vi "ecg_ncs_v9.vi"() -> ()   [LabVIEW 2016]
uses:
  <instrlib>/niUSRP/niUSRP Timestamp.ctl
  C:/Program Files/National Instruments/LabVIEW 2016/examples/Instrument IO/Serial/support/Serial - Settings.ctl
  State.ctl
  <vilib>/Instr/_visa.llb/VISA Configure Serial Port (Instr).vi
  <instrlib>/niUSRP/niUSRP Fetch Rx Data (2D CDB).vi
  <instrlib>/niUSRP/niUSRP Write Tx Data (2D CDB).vi
panel:
  out "#NCS Loops":i32
  out "size(s) 3":i32
  out "AmpNcsDSLast":dbl[](array[numeric])
  in  "Low-Pass Freq":dbl=200.0 format="%#_13g"
  in  "Wait  ECG":i32=2
  in  "max queue size":i32=-1
  in  "Wait NCS":i32=8
  out "ECG time":u32
  out "NCS time":u32
  in  "File Name 3":string="Test2"
  out "size(s) 4":i32
  in  "maxWrite 2":i32=2000
  out "AmpNcs":dbl[](array[numeric])
  out "PhNcs":dbl[](array[numeric])
  in  "Sampling Rate":i32=500
  out "AmpNcsDS":dbl[](array[numeric])
  out "PhNcsDS":dbl[](array[numeric])
  in  "Tab Control 3":enum32{"ECG Sample", "ECG"}(tab)
  out "?":i32(graph)
  out "?":i16(graph)
  in  "maxWrite":i32=2000
  out "size(s) 2":i32
  out "sizeNcsDS":i32
  in  "File Name":string="data"
  in  "Path":path=path "D:/Research/SummerFall17Spring18/CnC/NCS/EcgNcsCorrelation/CodeAndData/Data"
  out "#Loop = #Packets Received":i32
  out "ECGsample":i16
  out "error IO 2":errorcluster={"status"=FALSE, "code"=-1074118647, "source"=""}
  in  "Serial Settings":T1={"baud rate"=57600, "data bits"=8, "parity"=enum."None", "stop bits"=10, "flow control"=0} {"flow control" items=["None"=0, "XON/XOFF"=1, "RTS/CTS"=2, "DTR/DSR"=4]; "stop bits" items=["1.0"=10, "1.5"=15, "2.0"=20]; "data bits" min=5 max=8 step=1; "baud rate" items=["75"=75, "110"=110, "134"=134, "150"=150, "300"=300, "600"=600, "1200"=1200, "1800"=1800, "2400"=2400, "4800"=4800, "7200"=7200, "9600"=9600, "14400"=14400, "19200"=19200, "28800"=28800, "38400"=38400, "56000"=56000, "57600"=57600, "115200"=115200, "128000"=128000, "230400"=230400]}
  in  "VISA resource name":refnum<visa-resource-name>="bmd101"
  in  "byte count":u32=1
  out "Coerced Rx IQ Rate":dbl
  out "Gain":dbl=-15.0
  out "Bandwidth":dbl=56000000.0
  out "Coerced Carrier Frequency":dbl=2000000000.0 format="%#.17g"
  out "Coerced Tx IQ rate":dbl=1000000.0
  out "error IO":errorcluster={"status"=FALSE, "code"=-1074118647, "source"=""}
  in  "Rx Number of Samples":i32=2000
  in  "Tab Control 2":enum32{"NI-294x/295x", "NI-2900/2901"}(tab)=enum."NI-2900/2901"
  in  "Rx carrier frequency [Hz]":dbl=2000000000.0 format="%#_6p"
  in  "Tx carrier frequency [Hz]":dbl=1000000000.0 format="%#_6p"
  in  "Start Trigger Time":T2={"whole seconds"=1, "fractional seconds"=0.0}
  in  "Tab Control":T3(tab)
  out "?":dbl[](graph)
  out "NCS Amp Chart":dbl[](graph)=[0.011967714738528729, 0.012021355192189592, 0.012015275039596582, 0.011969166030167903, 0.011958890166168242, 0.012007893820858737, 0.012022893722444085, 0.011978222225113794, 0.011969989939463181, 0.012003099640895068]
  out "NCS Phase Chart":dbl[](graph)=[0.011967714738528729, 0.012021355192189592, 0.012015275039596582, 0.011969166030167903, 0.011958890166168242, 0.012007893820858737, 0.012022893722444085, 0.011978222225113794, 0.011969989939463181, 0.012003099640895068]
  out "Tx Waveform Graph":waveform(dbl)[](graph)
  in  "Stop":bool
  in  "Tone Amplitude":dbl=0.707 step=0.05 format="%#.6g"
  in  "Tone  Frequency":dbl=5000.0 format="%#_6p"
  in  "Tx Waveform Size":dbl=2000.0
  in  "Device Name":refnum<k15>="MyB210"
  in  "Tx Gain":dbl=28.0 format="%#_6f"
  in  "Tx IQ Rate":dbl=250000.0 format="%#_6p"
  in  "Rx Gain":dbl=32.0 format="%#_6f"
  in  "Rx IQ Rate":dbl=250000.0 format="%#_6p"
  # "Rx Settings"
  # "Tx Settings"
  # "Note that on the NI-2900 and NI-2901, both Rx channels share an LO and both Tx channels share an LO. However, on the NI-294x/295x devices, Rx and Tx of channel 0 share an LO and Rx and Tx of channel 1 share an LO."
  # "Rx: Number of samples should be 1e6/512 in one loop."
  # "This Tx graph should always have end and start tied up since this is being sent in a loop continuously. Otherwise phase jumps will be noticed."
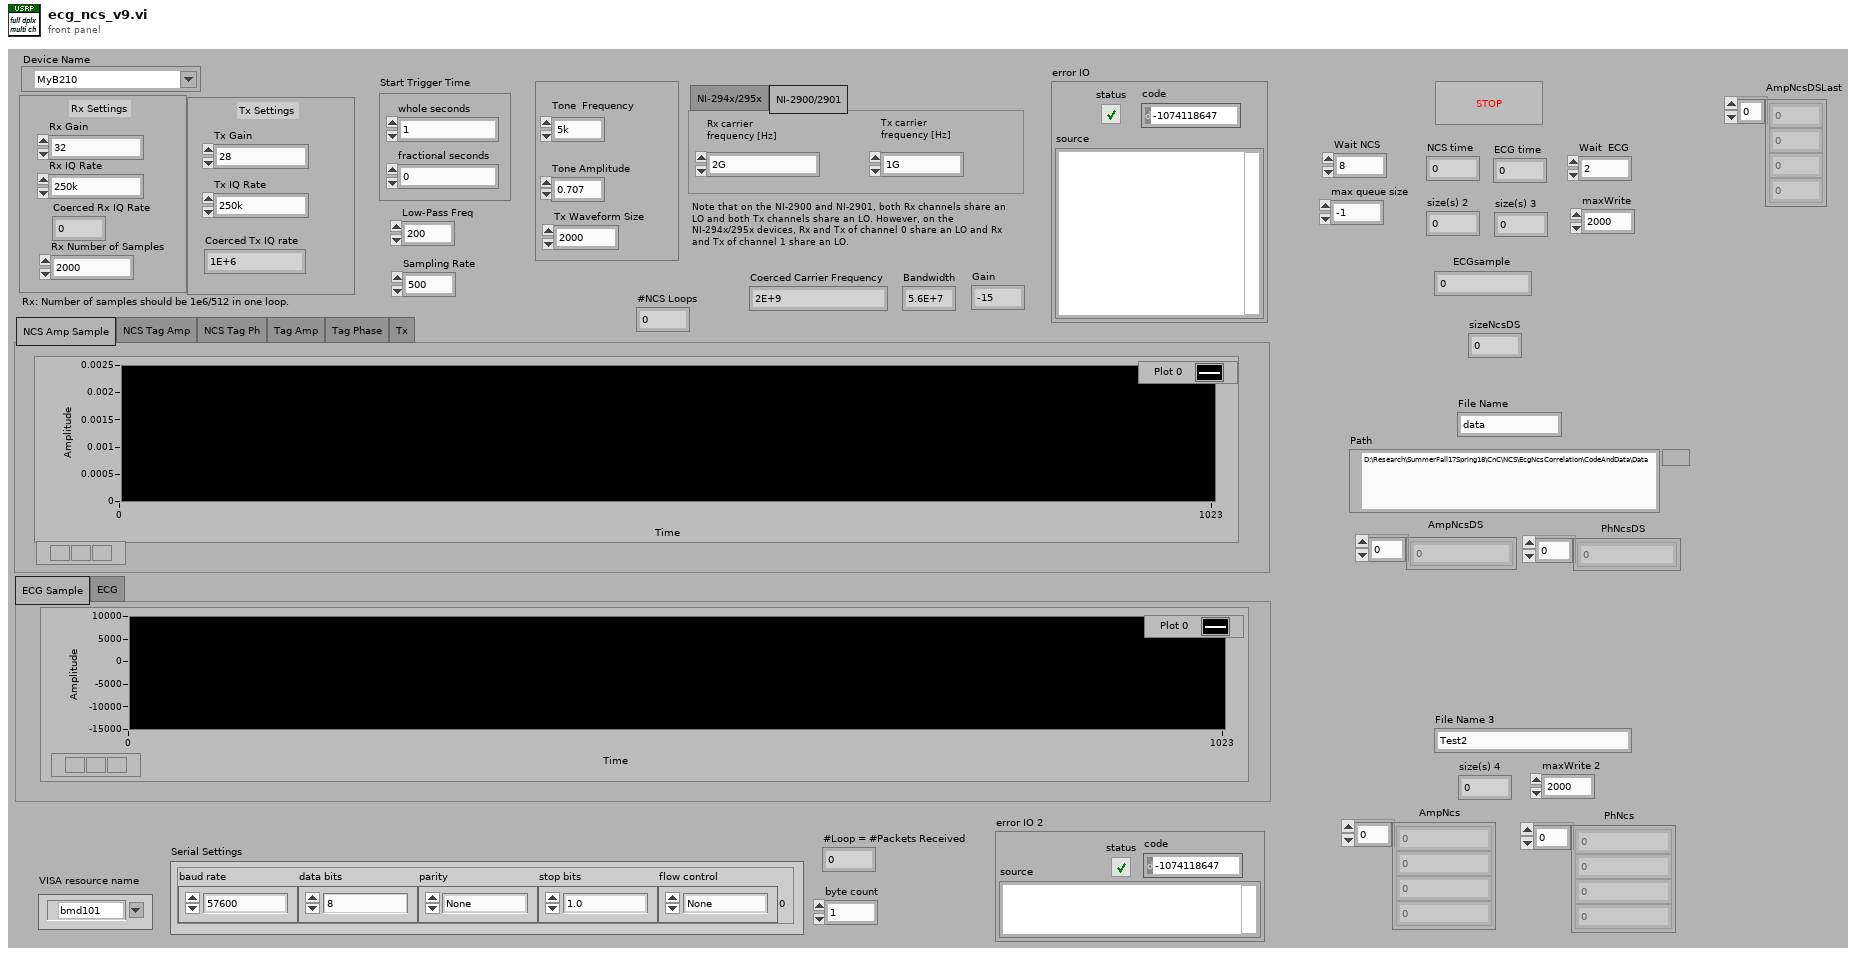
[diagram p1: front panel]
types:
  T1 = typedef "Serial - Settings.ctl" = cluster{"baud rate":u32, "data bits":u16, "parity":enum16{"None", "Odd", "Even", "Mark", "Space"}, "stop bits":u16, "flow control":u16}
  T2 = typedef "niUSRP Timestamp.ctl" = cluster{"whole seconds":u64, "fractional seconds":dbl}
  T3 = enum32{"NCS Amp Sample", "NCS Tag Amp", "NCS Tag Ph", "Tag Amp", "Tag Phase", "Tx"}
  T4 = typedef "State.ctl" = enum16{"Initialize", "get byte", "check", "packet received", "packet approved"}
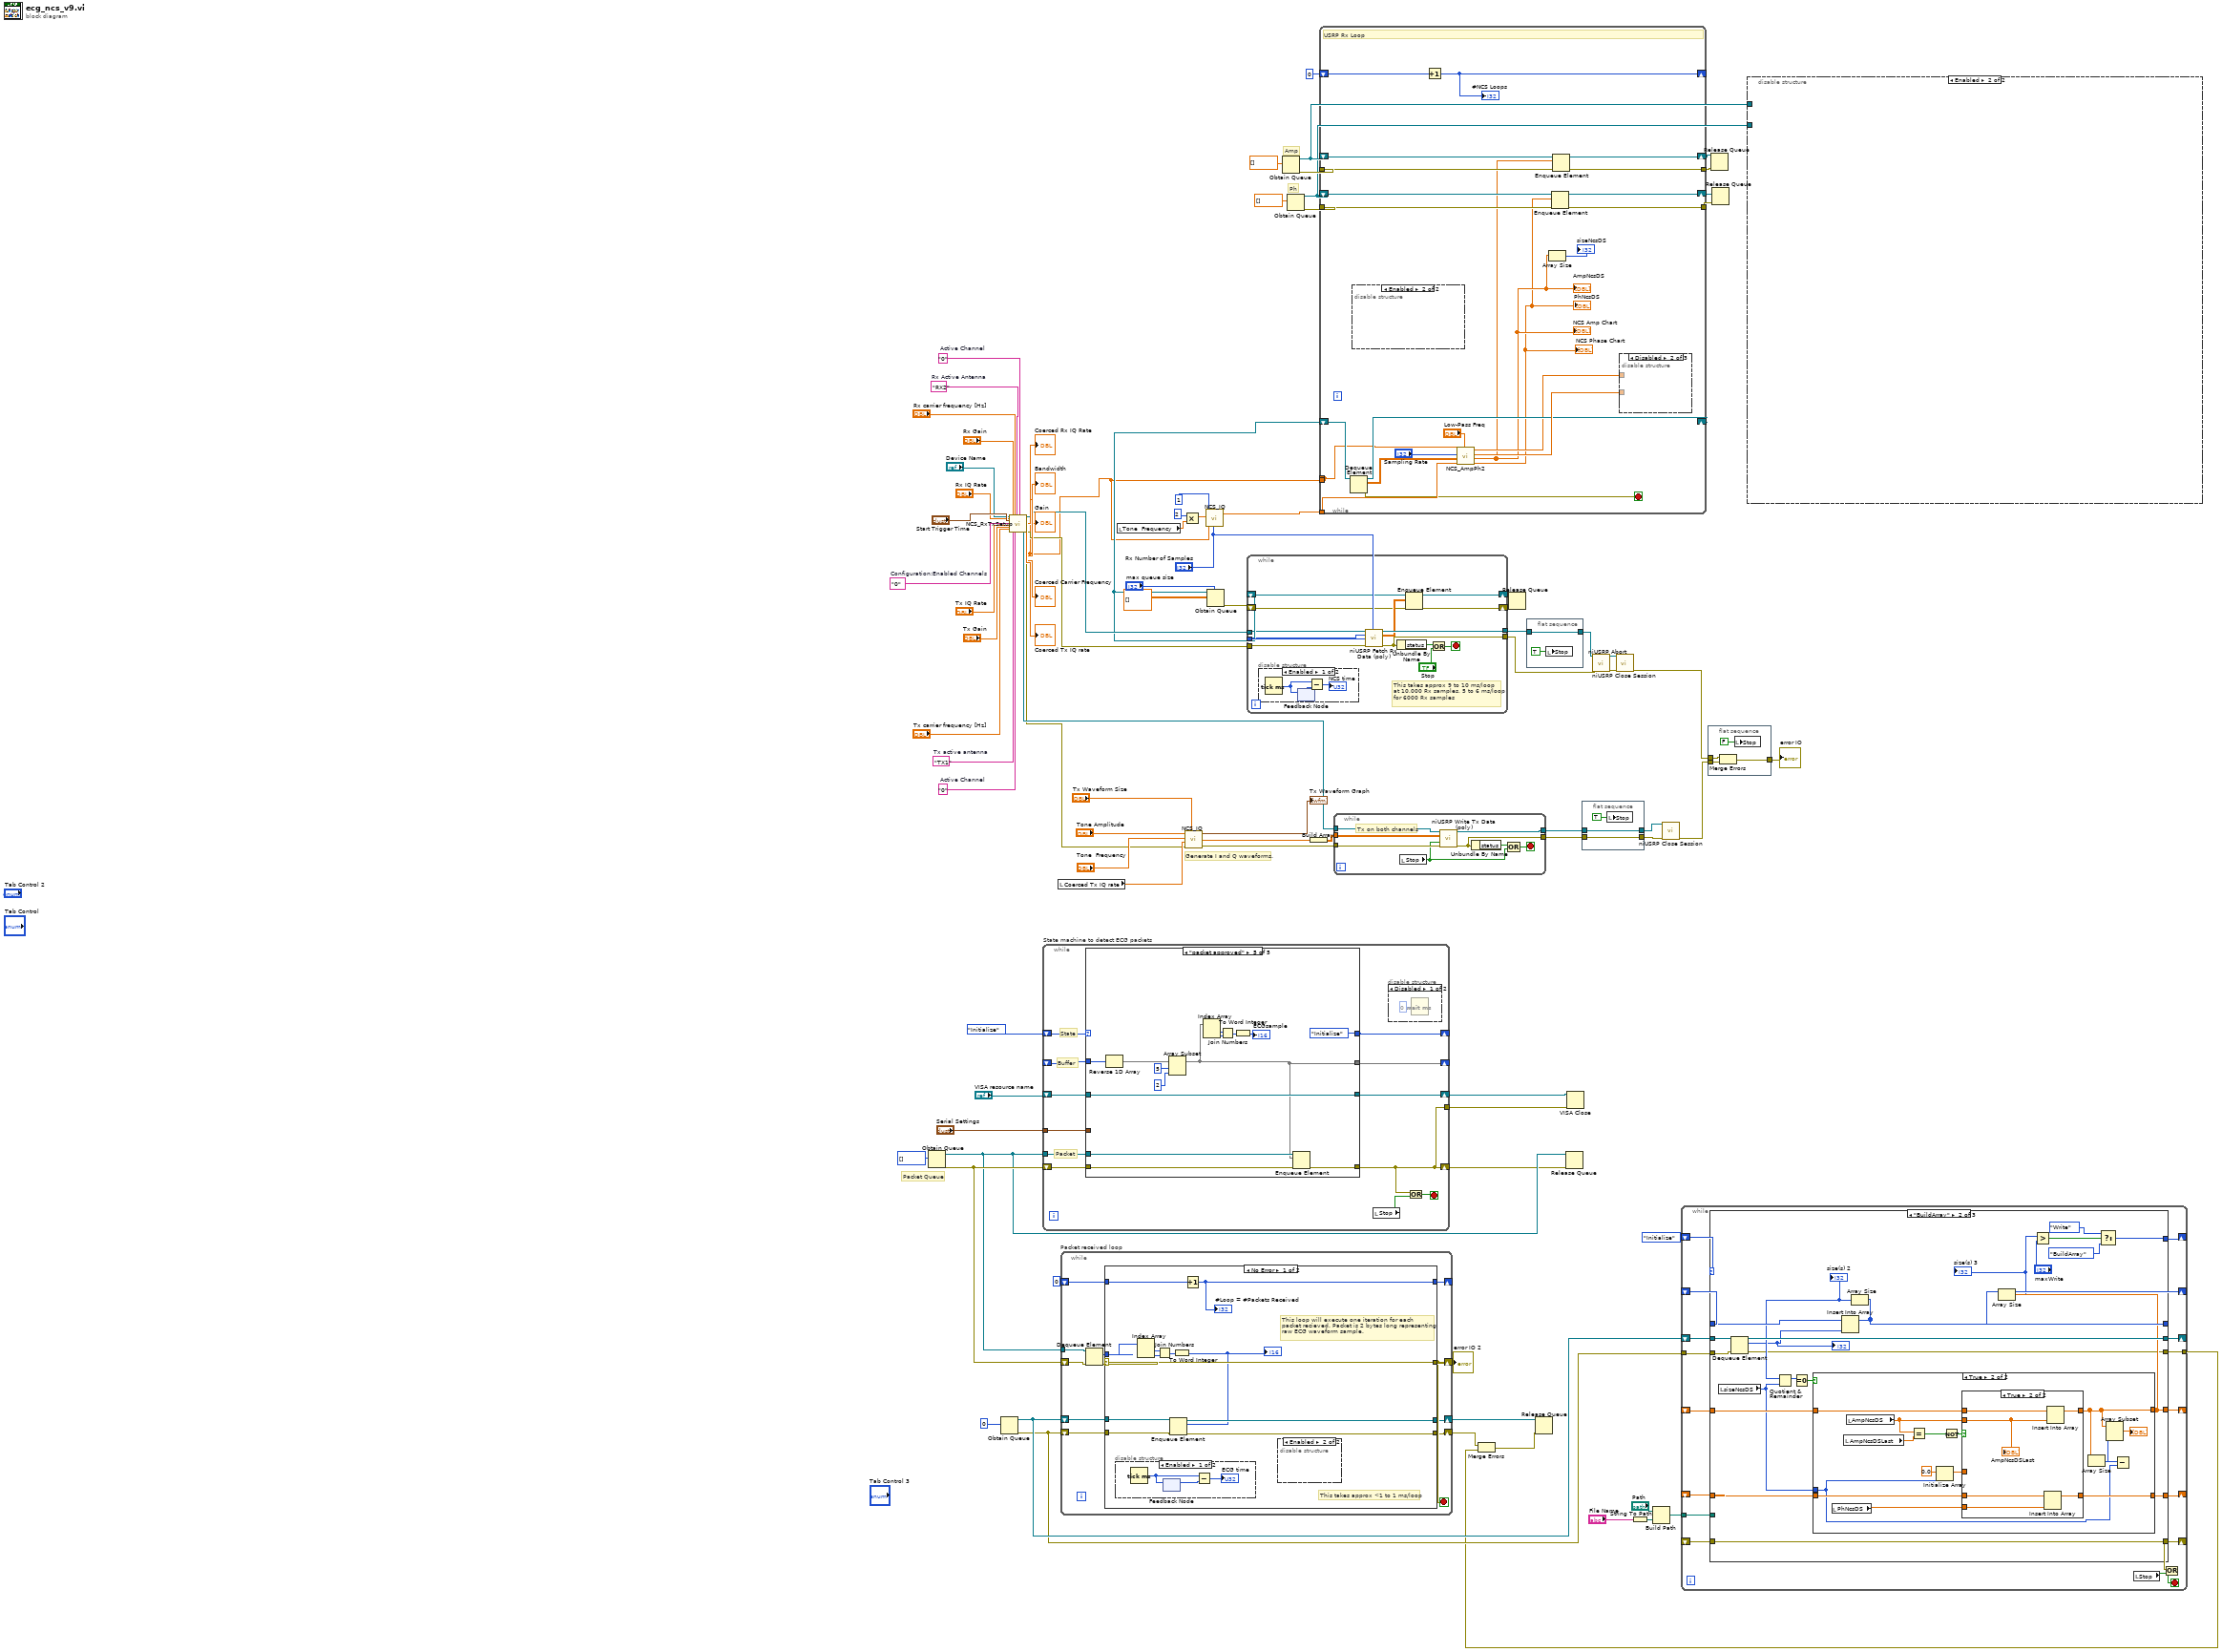
[diagram p0: block diagram]
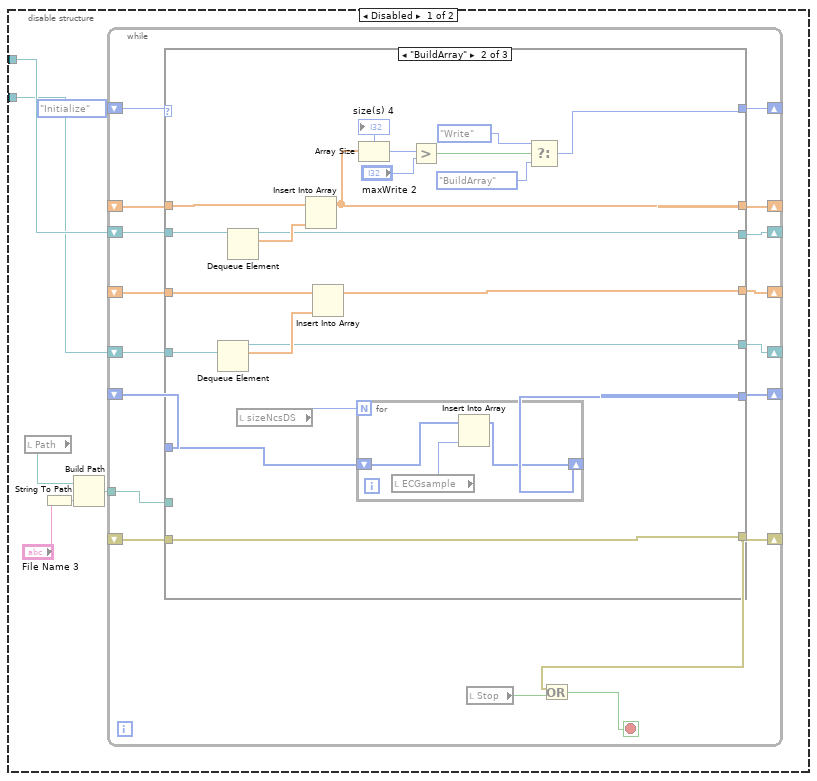
[diagram p2: hidden frame]
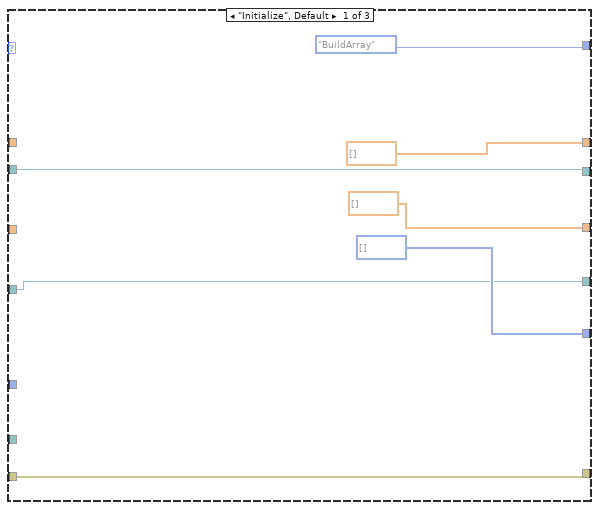
[diagram p3: hidden frame]
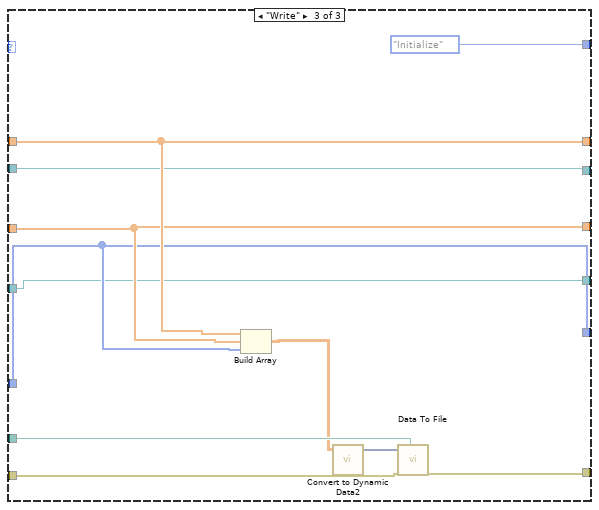
[diagram p4: hidden frame]
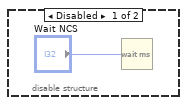
[diagram p5: hidden frame]
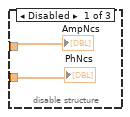
[diagram p6: hidden frame]
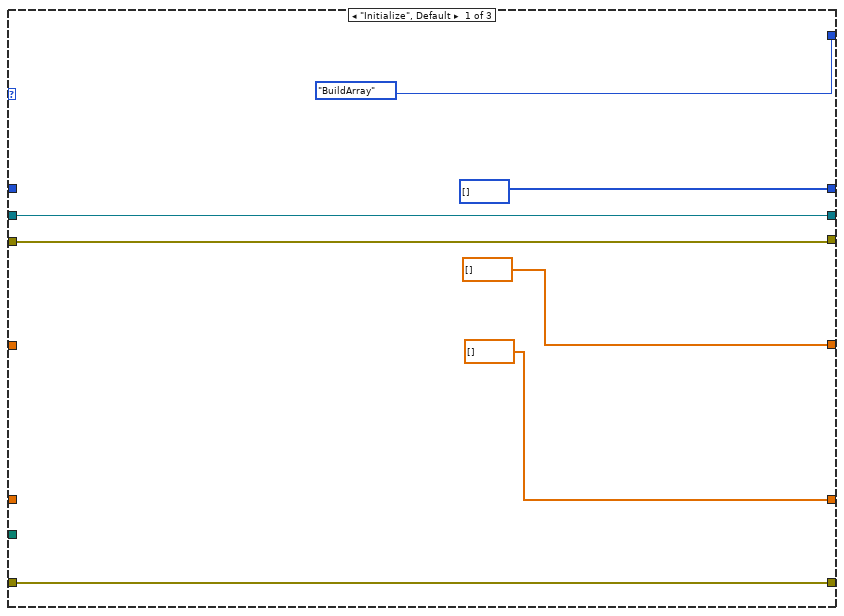
[diagram p8: hidden frame]
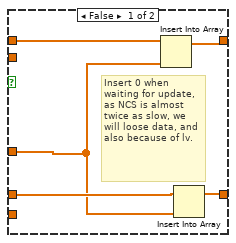
[diagram p10: hidden frame]
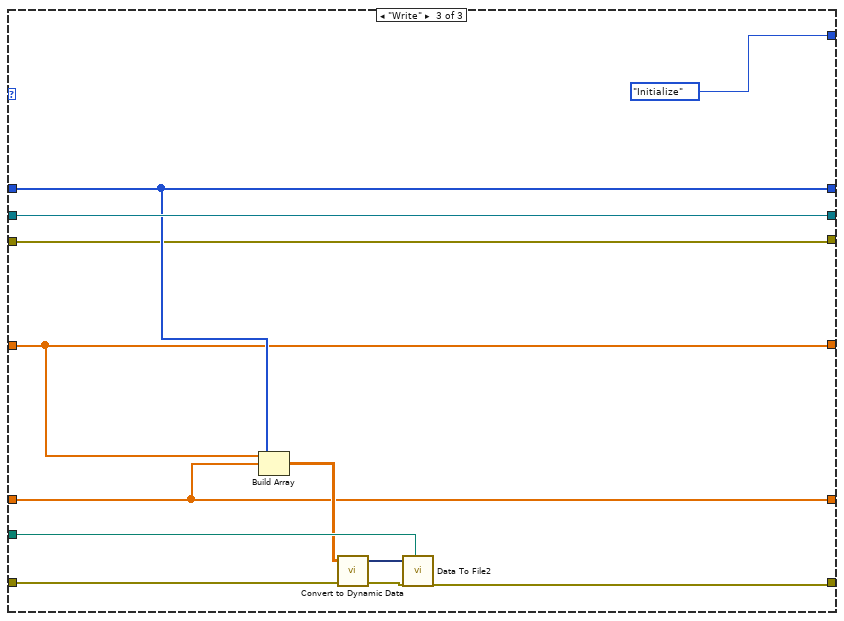
[diagram p11: hidden frame]
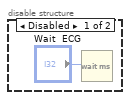
[diagram p13: hidden frame]
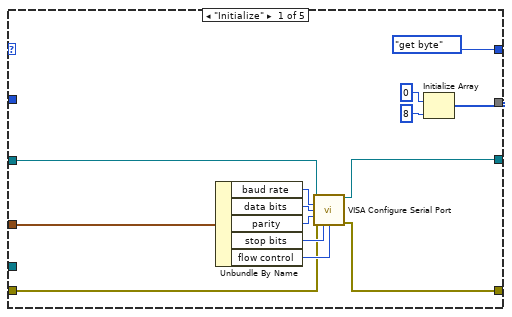
[diagram p17: hidden frame]
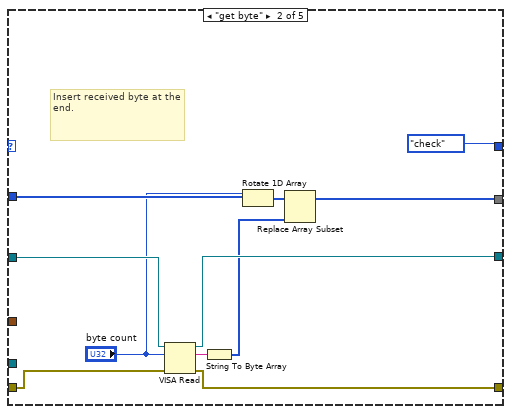
[diagram p18: hidden frame]
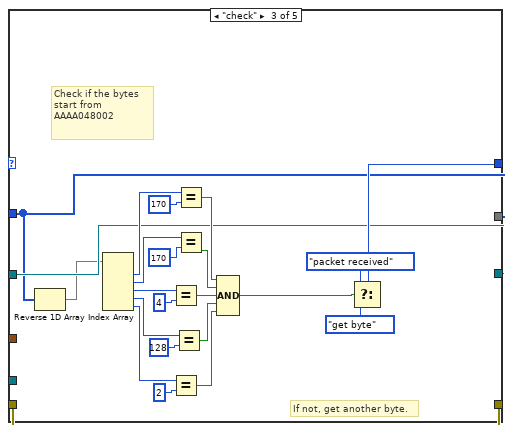
[diagram p19: hidden frame]
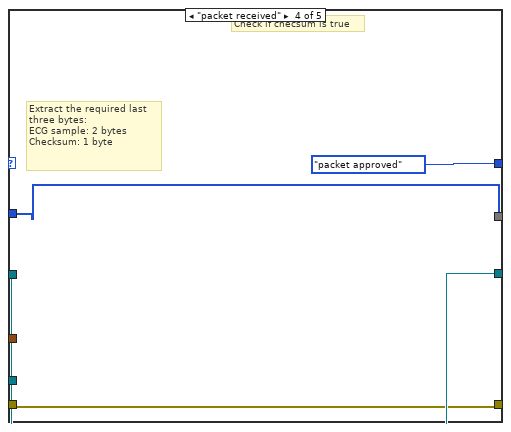
[diagram p20: hidden frame]
diagram:
  w50 = "0"  # Active Channel
  w51 = "0"  # Active Channel
  w80 = "RX2"  # Rx Active Antenna
  w76 = "TX1"  # Tx active antenna
  w65 = "0"  # Configuration:Enabled Channels
  # "Ph"
  # "Amp"
  # "Packet Queue"
  # "Generate I and Q waveforms."
  n1 = Obtain Queue(element data type=u8[] []) -> (queue out=w46:refnum<queue>, error out=w47:errorcluster)  [unwired: 4 in, 1 out]
  n2 = Obtain Queue(element data type=0) -> (queue out=w20:refnum<queue>, error out=w6:errorcluster)  [unwired: 4 in, 1 out]
  n3 = call "NCS_RxTxSetup.vi"("IVI Refnum in"="Device Name", "Rx IQ Rate"="Rx IQ Rate", "Start Trigger Time"="Start Trigger Time", "Configuration:Enabled Channels"=w65, "Tx IQ Rate"="Tx IQ Rate", "Tx Gain"="Tx Gain", "Tx carrier frequency [Hz]"="Tx carrier frequency [Hz]", "Rx Gain"="Rx Gain", "Tx active antenna"=w76, "Rx carrier frequency [Hz]"="Rx carrier frequency [Hz]", "Active Channel"=w50, "Rx Active Antenna"=w80, "Active Channel 2"=w51) -> ("session handle out"=w87:refnum<k15>, "IVI Refnum out"=w36:refnum<k15>, "Coerced Rx IQ Rate"=w8:dbl, "Bandwidth"=→"Bandwidth":dbl, "Gain"=→"Gain":dbl, "Carrier Frequency"=→"Coerced Carrier Frequency":dbl, "IQ Rate 2"=→"Coerced Tx IQ rate":dbl, "error out"=w37:errorcluster)  [unwired: 7 in]
  "Coerced Rx IQ Rate" <- w8
  n4 = while "State machine to detect ECG packets" {
    shift-right: [w90] -> w41
    shift-left: w47 -> [w96]
    shift-right: [w99] -> _
    shift-left: State."Initialize" ("State") -> [w98]
    shift-right: [w95] -> _
    shift-left: _ -> [w97]
    tunnel: w46 -> [w94]
    shift-right: [w93] -> w42
    shift-left: "VISA resource name" -> [w92]
    tunnel: "Serial Settings" -> [w91]
    tunnel: [w90] -> w40
    stop <- w89 stop-if-true
    # "State"
    # "Buffer"
    # "Packet"
    n5 = case shown="\"packet approved\"" w98 {
      tunnel: [w111 w123 w127 w150 w154] -> w95
      tunnel: [State."get byte" ("State") State."check" ("f") w147 State."packet approved" ("State") State."Initialize" ("State")] -> w99
      tunnel: w97 -> [_ w116 w127 w150 w159]
      tunnel: w96 -> [w105 w120 w148 w151 w162]
      tunnel: [w104 w119 w148 w151 w161] -> w90
      tunnel: w94 -> [_ _ _ _ w163]
      tunnel: [w103 w121 w128 w152 w160] -> w93
      tunnel: w92 -> [w102 w122 w128 w152 w160]
      tunnel: w91 -> [w101 _ _ _ _]
      frame "Initialize" {
        n6 = Unbundle By Name(w101) -> ("baud rate"=w110:u32, "data bits"=w109:u16, "parity"=w108:enum16{"None", "Odd", "Even", "Mark", "Space"}, "stop bits"=w107:u16, "flow control"=w106:u16)
        n7 = call-poly "VISA Configure Serial Port"("VISA resource name"=w102, "baud rate (9600)"=w110, "data bits (8)"=w109, "parity (0:none)"=w108, "error in (no error)"=w105, "stop bits (10: 1 bit)"=w107, "flow control (0:none)"=w106) -> ("VISA resource name out"=w103:refnum<visa-resource-name>, "error out"=w104:errorcluster)  [unwired: 3 in, 4 out]
        n8 = Initialize Array(u8 0, 8 ("dimension size")) -> (w111:u8[])
      }
      frame "get byte" {
        # "Insert received byte at the end."
        n9 = VISA Read(VISA resource name=w122, byte count="byte count", error in (no error)=w120) -> (VISA resource name out=w121:refnum<visa-resource-name>, read buffer=w118:string, error out=w119:errorcluster)  [unwired: 1 out]
        n10 = String To Byte Array(string=w118) -> (unsigned byte array=w117:u8[])
        n11 = Rotate 1D Array(1:w116, 2:"byte count") -> (0:w124:u8[])
        n12 = Replace Array Subset(array=w124, new element=w117) -> (w123:u8[])  [unwired: 1 in]
      }
      frame "check" {
        # "If not, get another byte."
        # "Check if the bytes start from AAAA048002"
        n13 = Reverse 1D Array(array=w127) -> (reversed array=w126:u8[])
        n14 = Index Array(array=w126) -> (element #1=w134:u8, element #2=w133:u8, element #3=w132:u8, element #4=w131:u8, element #5=w130:u8)  [unwired: 5 in]
        n15 = Equal?(x=w132, y=u8 4 ("element")) -> (x = y?=w137:bool)
        n16 = Equal?(x=w130, y=u8 2 ("element")) -> (x = y?=w135:bool)
        n17 = Equal?(x=w131, y=u8 128 ("element")) -> (x = y?=w136:bool)
        n18 = Equal?(x=w134, y=u8 170 ("element")) -> (x = y?=w139:bool)
        n19 = Equal?(x=w133, y=u8 170 ("element")) -> (x = y?=w138:bool)
        n20 = Compound Arithmetic op=AND(w139, w138, w137, w136, w135) -> (w129:bool)
        n21 = Select(t=State."packet received" ("f"), s=w129, f=State."get byte") -> (s? t:f=w147:T4)
      }
      frame "packet received" {
        # "Check if checsum is true"
        # "Extract the required last three bytes: \nECG sample: 2 bytes\nChecksum: 1 byte"
      }
      frame "packet approved" {
        n22 = Reverse 1D Array(array=w159) -> (reversed array=w158:u8[])
        n23 = Array Subset(array=w158, index=5, length=2 ("index")) -> (w154:u8[])
        n24 = Index Array(array=w154) -> (element #1=w157:u8, element #2=w156:u8)  [unwired: 2 in]
        n25 = Join Numbers(hi=w157, lo=w156) -> ((hi.lo)=w155:u16)
        n26 = To Word Integer(number=w155) -> (16bit integer=→"ECGsample":i16)
        n27 = Enqueue Element(queue=w163, element=w154, error in (no error)=w162) -> (error out=w161:errorcluster)  [unwired: 1 in, 2 out]
      }
    }
    n28 = local read "Stop"() -> (w88:bool)
    n29 = disable-structure shown="Disabled" {
      frame Disabled {
        n30 = Wait (ms)(milliseconds to wait=u32 0) -> ()  [unwired: 1 out]
      }
      frame Enabled {
      }
    }
    n31 = Or(x=w90, y=w88) -> (x .or. y?=w89:bool)
  }
  n32 = local read "Coerced Tx IQ rate"() -> (w60:dbl)
  n33 = while "Packet received loop" {
    shift-right: [w173] -> w43
    shift-left: w47 -> [w177]
    tunnel: w46 -> [w176]
    shift-right: [w171] -> _
    shift-left: 0 -> [w172]
    shift-right: [w168] -> w21
    shift-left: w20 -> [w170]
    shift-right: [w167] -> w5
    shift-left: w6 -> [w169]
    stop <- w173 stop-if-true
    n34 = Dequeue Element(queue=w176, error in (no error)=w177) -> (element=w175:u8[], error out=w174:errorcluster)  [unwired: 1 in, 2 out]
    n35 = case shown="No Error" w174 {
      selector: w174 -> [w183 w197]
      tunnel: w175 -> [w189 _]
      tunnel: [w183 w197] -> w173
      tunnel: w172 -> [w185 w196]
      tunnel: [w184 w196] -> w171
      tunnel: w170 -> [w182 w195]
      tunnel: w169 -> [w181 w194]
      tunnel: [w180 w195] -> w168
      tunnel: [w179 w194] -> w167
      frame No Error {
        # "This takes approx <1 to 1 ms/loop"
        # "This loop will execute one iteration for each\npacket recieved. Packet is 2 bytes long representing \nraw ECG waveform sample."
        n36 = disable-structure shown="Enabled" {
          frame Enabled {
            n37 = Tick Count (ms)() -> (millisecond timer value=w193:u32)
            n38 = feedback #1() -> (w192:u32)  [unwired: 1 in]
            n39 = feedback-in #1(w193) -> ()
            n40 = Subtract(x=w193, y=w192) -> (x-y=→"ECG time":u32)
          }
          frame Disabled {
          }
        }
        n41 = Index Array(array=w189) -> (element #1=w188:u8, element #2=w187:u8)  [unwired: 2 in]
        n42 = Join Numbers(hi=w188, lo=w187) -> ((hi.lo)=w186:u16)
        n43 = To Word Integer(number=w186) -> (16bit integer=w178:i16)
        "?" <- w178
        n44 = Enqueue Element(queue=w182, element=w178, error in (no error)=w181) -> (queue out=w180:refnum<queue>, error out=w179:errorcluster)  [unwired: 1 in, 1 out]
        n45 = Increment(x=w185) -> (x+1=w184:i32)
        "#Loop = #Packets Received" <- w184
        n46 = disable-structure shown="Enabled" {
          frame Disabled {
            n47 = Wait (ms)(milliseconds to wait="Wait  ECG") -> ()  [unwired: 1 out]
          }
          frame Enabled {
          }
        }
      }
      frame Error {
      }
    }
  }
  "error IO 2" <- w43
  n48 = local read "Tone  Frequency"() -> (w64:dbl)
  n49 = Multiply(x=2, y=w64) -> (x*y=w29:dbl)
  n50 = call "NCS_IQ.vi"("Tone Amplitude"="Tone Amplitude", "Waveform Size"="Tx Waveform Size", "Tone Frequency"="Tone  Frequency", "Coerced IQ rate"=w60, "error in (no error)"=w37) -> ("IQ waveform"=→"Tx Waveform Graph":waveform(dbl)[], "IQ waveform array"=w58:cdb[], "error out"=w59:errorcluster)  [unwired: 1 in]
  n51 = call "NCS_IQ.vi"("Tone Amplitude"=1, "Waveform Size"="Rx Number of Samples", "Tone Frequency"=w29, "Coerced IQ rate"=w8) -> ("IQ waveform array"=w7:cdb[])  [unwired: 2 in, 2 out]
  n52 = Obtain Queue(max queue size (-1, unlimited)="max queue size", element data type=dbl[][] []) -> (queue out=w9:refnum<queue>, error out=w33:errorcluster)  [unwired: 3 in, 1 out]
  n53 = while {
    tunnel: w37 -> [w210]
    tunnel: w36 -> [w209]
    tunnel: [w208] -> w35
    tunnel: [w200] -> w34
    shift-right: [w204] -> w32
    shift-left: w33 -> [w205]
    shift-right: [w203] -> w31
    shift-left: w9 -> [w207]
    tunnel: "Rx Number of Samples" -> [w202]
    stop <- w199 stop-if-true
    # "This takes approx 9 to 10 ms/loop\nat 10,000 Rx samples, 5 to 6 ms/loop \nfor 6000 Rx samples"
    n54 = disable-structure shown="Enabled" {
      frame Enabled {
        n55 = Tick Count (ms)() -> (millisecond timer value=w213:u32)
        n56 = feedback #2() -> (w212:u32)  [unwired: 1 in]
        n57 = feedback-in #2(w213) -> ()
        n58 = Subtract(x=w213, y=w212) -> (x-y=→"NCS time":u32)
      }
      frame Disabled {
      }
    }
    n59 = call-poly <instrlib>:"niUSRP Fetch Rx Data (poly).vi"("session handle"=w209, "number of samples"=w202, "error in (no error)"=w210) -> ("session handle out"=w208:refnum<k15>, "data"=w206:cdb[][], "error out"=w200:errorcluster)  [unwired: 9 in, 1 out]
    n60 = Unbundle By Name(w200) -> ("status"=w201:bool)
    n61 = Enqueue Element(queue=w207, element=w206, error in (no error)=w205) -> (queue out=w203:refnum<queue>, error out=w204:errorcluster)  [unwired: 1 in, 1 out]
    n62 = Or(x=w201, y="Stop") -> (x .or. y?=w199:bool)
  }
  n63 = Obtain Queue(element data type=dbl[] []) -> (queue out=w11:refnum<queue>, error out=w18:errorcluster)  [unwired: 4 in, 1 out]
  n64 = Obtain Queue(element data type=dbl[] []) -> (queue out=w10:refnum<queue>, error out=w12:errorcluster)  [unwired: 4 in, 1 out]
  n65 = Build Array(w58) -> (w84:cdb[][])
  n66 = while {
    tunnel: [w220] -> _
    shift-right: [w233] -> _
    shift-left: w9 -> [w234]
    tunnel: w7 -> [w231]
    shift-right: [w225] -> w17
    shift-left: w11 -> [w226]
    tunnel: w18 -> [w229]
    tunnel: [w228] -> w16
    shift-right: [w223] -> w14
    shift-left: w10 -> [w224]
    tunnel: [w222] -> w13
    tunnel: w12 -> [w221]
    tunnel: w8 -> [w220]
    shift-right: [w214] -> _
    shift-left: 0 -> [w215]
    stop <- w230 stop-if-true
    # "USRP Rx Loop"
    n67 = Dequeue Element(queue=w234) -> (queue out=w233:refnum<queue>, element=w232:dbl[][], error out=w230:errorcluster)  [unwired: 2 in, 1 out]
    n68 = disable-structure shown="Enabled" {
      frame Disabled {
        n69 = Wait (ms)(milliseconds to wait="Wait NCS") -> ()  [unwired: 1 out]
      }
      frame Enabled {
      }
    }
    n70 = Increment(x=w215) -> (x+1=w214:i32)
    "#NCS Loops" <- w214
    n71 = call "NCS_AmpPh2.vi"("Low-Pass Freq"="Low-Pass Freq", "IQ"=w231, "data"=w232, "Sampling Rate"="Sampling Rate", "Coerced Rx IQ Rate"=w220) -> ("Phase DownSampled"=w217:dbl[], "Amp DownSampled"=w218:dbl[], "Phase"=w235:dbl[], "Amplitude"=w227:dbl[])  [unwired: 2 in, 1 out]
    "AmpNcsDS" <- w218
    "PhNcsDS" <- w217
    "NCS Amp Chart" <- w218
    "NCS Phase Chart" <- w217
    n72 = Array Size(array=w218) -> (size(s)=→"sizeNcsDS":i32)
    n73 = Enqueue Element(queue=w224, element=w217, error in (no error)=w221) -> (queue out=w223:refnum<queue>, error out=w222:errorcluster)  [unwired: 1 in, 1 out]
    n74 = Enqueue Element(queue=w226, element=w218, error in (no error)=w229) -> (queue out=w225:refnum<queue>, error out=w228:errorcluster)  [unwired: 1 in, 1 out]
    n75 = disable-structure shown="Disabled" {
      disable-tunnel: w227 -> [w238 _ _]
      disable-tunnel: w235 -> [w239 _ _]
      frame Disabled {
        "AmpNcs" <- w238
        "PhNcs" <- w239
      }
      frame Disabled {
      }
      frame Enabled {
      }
    }
  }
  n76 = while {
    tunnel: w87 -> [w247]
    tunnel: w59 -> [w246]
    tunnel: [w244] -> w75
    tunnel: [w242] -> w71
    tunnel: w84 -> [w240]
    stop <- w243 stop-if-true
    # "Tx on both channels"
    n77 = local read "Stop"() -> (w241:bool)
    n78 = call-poly <instrlib>:"niUSRP Write Tx Data (poly).vi"("session handle"=w247, "data"=w240, "end of data?"=w241, "error in (no error)"=w246) -> ("session handle out"=w242:refnum<k15>, "error out"=w244:errorcluster)  [unwired: 10 in]
    n79 = Unbundle By Name(w244) -> ("status"=w245:bool)
    n80 = Compound Arithmetic op=OR(w245, w241) -> (w243:bool)
  }
  n81 = Release Queue(queue=w31, error in (no error)=w32) -> ()  [unwired: 1 in, 3 out]
  n82 = flat-sequence {
    tunnel: [w248] -> w73
    tunnel: w35 -> [w248]
    frame #0 {
      n83 = local write "Stop"(TRUE ("STOP")) -> ()
    }
  }
  n84 = Release Queue(queue=w46, error in (no error)=w41) -> ()  [unwired: 1 in, 3 out]
  n85 = VISA Close(VISA resource name=w42, error in (no error)=w40) -> ()  [unwired: 1 out]
  n86 = flat-sequence {
    tunnel: [w251] -> w74
    tunnel: w75 -> [w251]
    tunnel: [w250] -> w72
    tunnel: w71 -> [w250]
    frame #0 {
      n87 = local write "Stop"(TRUE ("STOP")) -> ()
    }
  }
  n88 = call <instrlib>:"niUSRP Abort.vi"("session handle"=w73, "error in (no error)"=w34) -> ("session handle out"=w86:refnum<k15>, "error out"=w85:errorcluster)  [unwired: 12 in]
  n89 = call <instrlib>:"niUSRP Close Session.vi"("session handle"=w86, "error in (no error)"=w85) -> ("error out"=w68:errorcluster)  [unwired: 13 in]
  n90 = String To Path(string="File Name") -> (path=w27:path)
  n91 = Build Path(base path="Path", name or relative path=w27) -> (appended path=w23:path)
  n92 = call <instrlib>:"niUSRP Close Session.vi"("session handle"=w72, "error in (no error)"=w74) -> ("error out"=w70:errorcluster)  [unwired: 13 in]
  n93 = while {
    shift-right: [w268] -> _
    shift-left: _ -> [w269]
    shift-right: [w266] -> _
    shift-left: _ -> [w267]
    shift-right: [w264] -> _
    shift-left: enum16{"Initialize", "BuildArray", "Write"}."Initialize" -> [w265]
    tunnel: w23 -> [w263]
    shift-right: [w260] -> _
    shift-left: _ -> [w259]
    shift-right: [w257] -> _
    shift-left: w20 -> [w258]
    shift-right: [w256] -> _
    shift-left: _ -> [w255]
    tunnel: w6 -> [w254]
    tunnel: [w253] -> w4
    stop <- w261 stop-if-true
    n94 = case shown="\"BuildArray\"" w265 {
      tunnel: w269 -> [_ w298 w330]
      tunnel: [i32[] [] w296 w330] -> w268
      tunnel: w267 -> [_ w297 w328]
      tunnel: [dbl[] [] w286 w328] -> w266
      tunnel: [enum16{"Initialize", "BuildArray", "Write"}."BuildArray" w291 enum16{"Initialize", "BuildArray", "Write"}."Initialize"] -> w264
      tunnel: w263 -> [_ _ w335]
      tunnel: [w275 w290 w333] -> w260
      tunnel: w259 -> [w275 w290 w332]
      tunnel: w258 -> [w274 w289 w331]
      tunnel: [w274 w288 w331] -> w257
      tunnel: [dbl[] [] w282 w329] -> w256
      tunnel: w255 -> [_ w287 w329]
      tunnel: w254 -> [w270 w279 w327]
      tunnel: [w270 w278 w327] -> w253
      frame "Initialize", Default {
      }
      frame "BuildArray" {
        n95 = local read "sizeNcsDS"() -> (w277:i32)
        n96 = Dequeue Element(queue=w289, error in (no error)=w279) -> (queue out=w288:refnum<queue>, element=w280:i32, error out=w278:errorcluster)  [unwired: 1 in, 1 out]
        "?" <- w280
        n97 = Insert Into Array(array=w298, new element=w280) -> (w296:i32[])  [unwired: 1 in]
        n98 = Array Size(array=w296) -> (size(s)=w285:i32)
        "size(s) 2" <- w285
        n99 = Quotient & Remainder(x=w285, y=w277) -> (x-y*floor(x/y)=w284:i32)  [unwired: 1 out]
        n100 = Equal To 0?(x=w284) -> (x = 0?=w283:bool)
        n101 = case shown="True" w283 {
          tunnel: w297 -> [w299 w315]
          tunnel: [w299 w314] -> w286
          tunnel: w287 -> [w300 w312]
          tunnel: [w300 w306] -> w282
          tunnel: w277 -> [_ w302]
          frame False {
          }
          frame True {
            n102 = local read "PhNcsDS"() -> (w313:dbl[])
            n103 = local read "AmpNcsDSLast"() -> (w301:dbl[])
            n104 = local read "AmpNcsDS"() -> (w311:dbl[])
            n105 = Equal?(x=w311, y=w301) -> (x = y?=w310:bool)
            n106 = Initialize Array(0.0 ("element"), w302) -> (w307:dbl[])
            n107 = Not(x=w310) -> (.not. x?=w309:bool)
            n108 = case shown="True" w309 {
              tunnel: w312 -> [w320 w326]
              tunnel: w315 -> [w318 w325]
              tunnel: [w317 w324] -> w314
              tunnel: w313 -> [_ w323]
              tunnel: w311 -> [_ w322]
              tunnel: [w319 w321] -> w306
              tunnel: w307 -> [w316 _]
              frame False {
                # "Insert 0 when \nwaiting for update,\nas NCS is almost \ntwice as slow, we \nwill loose data, and also because of lv."
                n109 = Insert Into Array(array=w320, new element=w316) -> (w319:dbl[])  [unwired: 1 in]
                n110 = Insert Into Array(array=w318, new element=w316) -> (w317:dbl[])  [unwired: 1 in]
              }
              frame True {
                n111 = Insert Into Array(array=w325, new element=w323) -> (w324:dbl[])  [unwired: 1 in]
                n112 = Insert Into Array(array=w326, new element=w322) -> (w321:dbl[])  [unwired: 1 in]
                "AmpNcsDSLast" <- w322
              }
            }
            n113 = Array Size(array=w306) -> (size(s)=w305:i32)
            n114 = Subtract(x=w305, y=w302) -> (x-y=w303:i32)
            n115 = Array Subset(array=w306, index=w303) -> (→"?":dbl[])  [unwired: 1 in]
          }
        }
        n116 = Array Size(array=w282) -> (size(s)=w281:i32)
        "size(s) 3" <- w281
        n117 = Greater?(x=w281, y="maxWrite") -> (0:w294:bool)
        n118 = Select(t=enum16{"Initialize", "BuildArray", "Write"}."Write", s=w294, f=enum16{"Initialize", "BuildArray", "Write"}."BuildArray") -> (s? t:f=w291:enum16{"Initialize", "BuildArray", "Write"})
      }
      frame "Write" {
        n119 = Build Array(w329, w328, w330) -> (w334:dbl[][])
        n120 = call "Convert to Dynamic Data"("2D Array"=w334) -> ("Dynamic Data Type"=w336:dynamicdata)  [unwired: 3 in]
        n121 = call "Data To File2"("Signals"=w336, "error in (no error)"=w332, "Filename"=w335) -> ("error out"=w333:errorcluster)  [unwired: 14 in, 2 out]
      }
    }
    n122 = local read "Stop"() -> (w262:bool)
    n123 = Or(x=w260, y=w262) -> (x .or. y?=w261:bool)
  }
  n124 = Merge Errors(w5, w4) -> (w3:errorcluster)
  n125 = Release Queue(queue=w21, error in (no error)=w3) -> ()  [unwired: 1 in, 3 out]
  n126 = flat-sequence {
    tunnel: w70 -> [w340]
    tunnel: [w339] -> w69
    tunnel: w68 -> [w338]
    frame #0 {
      n127 = Merge Errors(w338, w340) -> (w339:errorcluster)
      n128 = local write "Stop"(FALSE ("STOP")) -> ()
    }
  }
  n129 = Release Queue(queue=w17, error in (no error)=w16) -> ()  [unwired: 1 in, 3 out]
  n130 = Release Queue(queue=w14, error in (no error)=w13) -> ()  [unwired: 1 in, 3 out]
  n131 = disable-structure shown="Enabled" {
    disable-tunnel: w11 -> [w344 _]
    disable-tunnel: w10 -> [w343 _]
    frame Disabled {
      n132 = local read "Path"() -> (w342:path)
      n133 = String To Path(string="File Name 3") -> (path=w348:path)
      n134 = Build Path(base path=w342, name or relative path=w348) -> (appended path=w345:path)
      n135 = while {
        shift-right: [w364] -> _
        shift-left: _ -> [w365]
        shift-right: [w360] -> _
        shift-left: _ -> [w363]
        shift-right: [w361] -> _
        shift-left: _ -> [w362]
        shift-right: [w358] -> _
        shift-left: enum16{"Initialize", "BuildArray", "Write"}."Initialize" -> [w359]
        tunnel: w345 -> [w357]
        shift-right: [w354] -> _
        shift-left: _ -> [w353]
        shift-right: [w351] -> _
        shift-left: w344 -> [w352]
        shift-right: [w349] -> _
        shift-left: w343 -> [w350]
        stop <- w355 stop-if-true
        n136 = case shown="\"BuildArray\"" w359 {
          tunnel: w365 -> [_ w392 w403]
          tunnel: [dbl[] [] w387 w403] -> w364
          tunnel: w363 -> [_ w391 w402]
          tunnel: w362 -> [_ w390 w401]
          tunnel: [i32[] [] w389 w401] -> w361
          tunnel: [dbl[] [] w388 w402] -> w360
          tunnel: [enum16{"Initialize", "BuildArray", "Write"}."BuildArray" w381 enum16{"Initialize", "BuildArray", "Write"}."Initialize"] -> w358
          tunnel: w357 -> [_ _ w404]
          tunnel: [w368 w380 w399] -> w354
          tunnel: w353 -> [w368 w380 w398]
          tunnel: w352 -> [w367 w378 w397]
          tunnel: [w367 w377 w397] -> w351
          tunnel: w350 -> [w366 w376 w396]
          tunnel: [w366 w374 w396] -> w349
          frame "Initialize", Default {
          }
          frame "BuildArray" {
            n137 = Dequeue Element(queue=w376) -> (queue out=w374:refnum<queue>, element=w375:dbl[])  [unwired: 2 in, 2 out]
            n138 = Dequeue Element(queue=w378) -> (queue out=w377:refnum<queue>, element=w379:dbl[])  [unwired: 2 in, 2 out]
            n139 = local read "sizeNcsDS"() -> (w373:i32)
            n140 = Insert Into Array(array=w392, new element=w379) -> (w387:dbl[])  [unwired: 1 in]
            n141 = Insert Into Array(array=w391, new element=w375) -> (w388:dbl[])  [unwired: 1 in]
            n142 = for {
              N: w373 -> [_]
              shift-right: [w393] -> w389
              shift-left: w390 -> [w394]
              n143 = local read "ECGsample"() -> (w395:i16)
              n144 = Insert Into Array(array=w394, new element=w395) -> (w393:i32[])  [unwired: 1 in]
            }
            n145 = Array Size(array=w387) -> (size(s)=w386:i32)
            "size(s) 4" <- w386
            n146 = Greater?(x=w386, y="maxWrite 2") -> (0:w384:bool)
            n147 = Select(t=enum16{"Initialize", "BuildArray", "Write"}."Write", s=w384, f=enum16{"Initialize", "BuildArray", "Write"}."BuildArray") -> (s? t:f=w381:enum16{"Initialize", "BuildArray", "Write"})
          }
          frame "Write" {
            n148 = Build Array(w403, w402, w401) -> (w400:dbl[][])
            n149 = call "Convert to Dynamic Data2"("2D Array"=w400) -> ("Dynamic Data Type"=w405:dynamicdata)  [unwired: 3 in]
            n150 = call "Data To File"("Signals"=w405, "error in (no error)"=w398, "Filename"=w404) -> ("error out"=w399:errorcluster)  [unwired: 14 in, 2 out]
          }
        }
        n151 = local read "Stop"() -> (w356:bool)
        n152 = Or(x=w354, y=w356) -> (x .or. y?=w355:bool)
      }
    }
    frame Enabled {
    }
  }
  "error IO" <- w69
